vi "testSignal.vi"() -> ()   [LabVIEW 2014]
panel:
  out "Filtered Signal":dynamicdata(graph)
  out "Triggered Signals":dynamicdata(graph)
  in  "Frequency":dbl=10.1
  in  "Amplitude":dbl=1.0
  out "Sine":dynamicdata(graph)
  in  "stop":bool
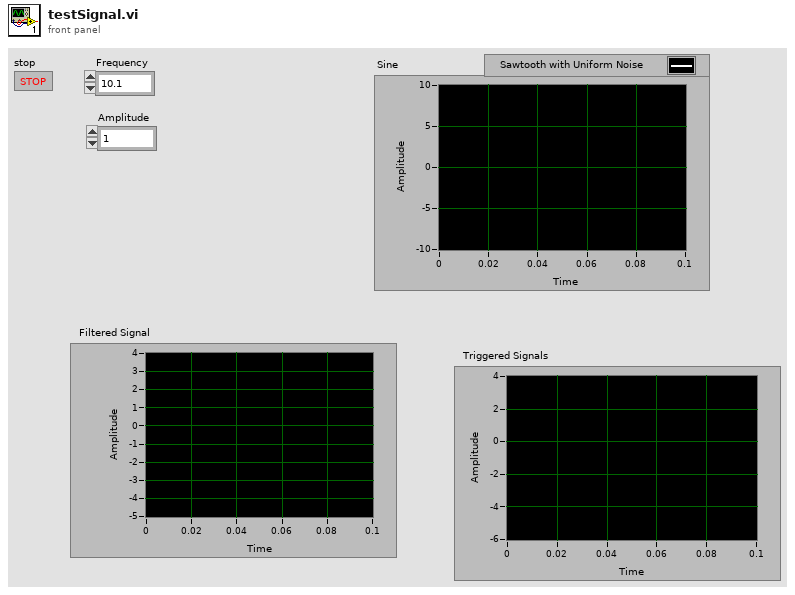
[diagram p1: front panel]
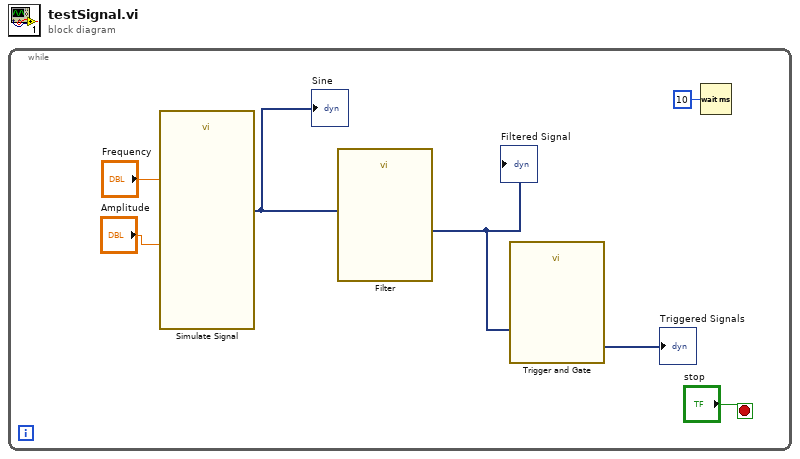
[diagram p0: block diagram]
diagram:
  n1 = while {
    stop <- "stop" stop-if-true
    n2 = call "Simulate Signal"("Frequency"="Frequency", "Amplitude"="Amplitude") -> ("Sawtooth with Uniform Noise"=w2:dynamicdata)  [unwired: 12 in, 1 out]
    "Sine" <- w2
    n3 = call "Filter"("Signal"=w2) -> ("Filtered Signal"=w1:dynamicdata)  [unwired: 9 in, 1 out]
    "Filtered Signal" <- w1
    n4 = call "Trigger and Gate"("Signals"=w1) -> ("Triggered Signals"=→"Triggered Signals":dynamicdata)  [unwired: 7 in, 3 out]
    n5 = Wait (ms)(milliseconds to wait=u32 10) -> ()  [unwired: 1 out]
  }
